vi "DSF.Engine.Builder.Get Plugins.vi"(11 "Builder in":refnum<class "DSF.Engine.Builder.lvclass">) -> (2 "Plugins":refnum<class "Plugin.lvclass">[](array[class]), 3 "Builder out":refnum<class "DSF.Engine.Builder.lvclass">)   [LabVIEW 2016, in "DSF.Engine.lvlib" / "DSF.Engine.Builder.lvclass"]
uses:
  DSF.Engine.Builder.lvclass
  Plugin/Plugin.lvclass
  DSF.Engine.Builder.lvclass/DSF.Engine.Builder.ctl
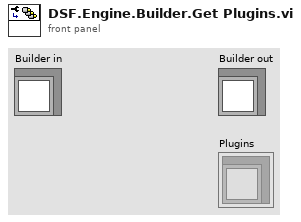
[diagram p1: front panel]
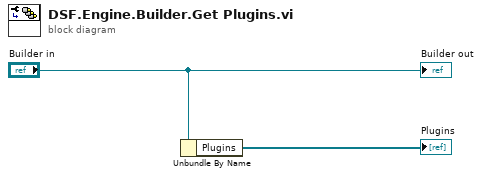
[diagram p0: block diagram]
diagram:
  n1 = Unbundle By Name("Builder in") -> ("Plugins"=→"Plugins":refnum<class "Plugin.lvclass">[])
  "Builder out" <- "Builder in"
